vi "Client Init Test.vi"() -> (0 "no error":errorcluster, 1 "tags found":bool, 2 "expected execution settings":bool)   [LabVIEW 2013, in "OPC UA Server tests.lvlib"]
doc: "Tests Init override for server configuration"
uses:
  OPC UA Server tests.lvlib
  module/execution/OPC UA Server runtime.lvclass
  <vilib>/OPCUA/server/subVI/supported security policies.ctl
  module/configuration/OPC UA Server configuration.lvclass
  module/configuration/OPC UA Server configuration.lvclass/OPC UA Server configuration.ctl
  <vilib>/NI/Tag Bus/tag/tag descriptor.lvclass/tag descriptor.ctl
  <vilib>/NI/Tag Bus Module Framework/channel/TBM channel.lvclass/TBM channel.ctl
  <vilib>/NI/Tag Bus/tag/read tag name.vi
  <vilib>/NI/Tag Bus/tag/read data type.vi
  <vilib>/NI/Tag Bus Module Framework/channel/Read channel classification.vi
  module/configuration/Read Lines.vi
  <vilib>/NI/Tag Bus/dictionary/data dictionary.lvclass
  <vilib>/NI/Tag Bus Module Framework/channel/TBM channel.lvclass
  <vilib>/opcua/NI OPC UA Server.lvlib
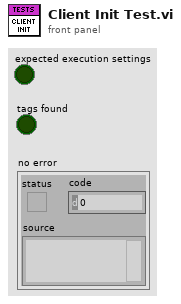
[diagram p1: front panel]
types:
  T1 = typedef "supported security policies.ctl" = cluster{"None":bool, "Sign with Basic128Rsa125":bool, "Sign and Encrypt with Basic128Rsa125":bool, "Sign with Basic256":bool, "Sign and Encrypt with Basic256":bool}
  T2 = cluster{"Client?":bool, "Server Certificates":cluster{"Relative Path?":bool, "Certificate Paths":path[], "Certificate Names":string[]}, "Client Certificates":cluster{"Relative Path?":bool, "Certificate Paths":path[], "Certificate Names":string[]}, "Client Configuration":cluster{"Server Endpoint URL":string, "Security Policy":cluster{"Message Mode":enum16{"None", "Sign", "Sign and Encrypt"}, "Security":enum16{"Basic256", "Basic128Rsa15"}}, "Username/Password":cluster{"Username":string, "Password":string}}, "Server Configuration":cluster{"Server Name":string, "TCP port (49580)":string, "Supported Security Policies":T1}}
  T3 = typedef "OPC UA configuration.lvclass/Line.ctl" = cluster{"channel":refnum<class "TBM channel.lvclass">, "Node Path":string, "OPC UA Data Type":T4}
  T4 = typedef "OPC UA configuration.lvclass/OPC UA Data Type.ctl" = u16
  T5 = typedef "TBM channel.lvclass/data tables.ctl" = cluster{"input data":T6, "processing parameter":T6, "processing result":T6, "output data":T6}
  T6 = typedef "tag bus.lvlib/dictionary table pair.ctl" = cluster{"data dictionary":refnum<class "data dictionary.lvclass">, "data table":T7}
  T7 = typedef "tag bus.lvlib/data table.lvlib/data table.ctl" = cluster{"Double":dbl[], "Single":sgl[], "I64":i64[], "I32":i32[], "I16":i16[], "I8":i8[], "U64":u64[], "U32":u32[], "U16":u16[], "U8":u8[], "Boolean":bool[], "String":string[], "Array of Double":cluster{"DBL Array":dbl[]}[], "Array of Single":cluster{"SGL Array":sgl[]}[], "Array of I64":cluster{"I64 Array":i64[]}[], "Array of I32":cluster{"I32 Array":i32[]}[], "Array of I16":cluster{"I16 Array":i16[]}[], "Array of I8":cluster{"I8 Array":i8[]}[], "Array of U64":cluster{"U64 Array":u64[]}[], "Array of U32":cluster{"U32 Array":u32[]}[], "Array of U16":cluster{"U16 Array":u16[]}[], "Array of U8":cluster{"U8 Array":u8[]}[], "Array of Boolean":cluster{"Boolean Array":bool[]}[], "Array of String":cluster{"String Array":string[]}[]}
  T8 = typedef "TBM module execution interface.lvclass/execution settings.ctl" = cluster{"reads inputs":bool, "processes data":bool, "writes outputs":bool}
  T9 = typedef "tag bus.lvlib/tag descriptor.lvclass/Data Type.ctl" = enum16{"Double", "Single", "I64", "I32", "I16", "I8", "U64", "U32", "U16", "U8", "Boolean", "String", "Array of Double", "Array of Single", "Array of I64", "Array of I32", "Array of I16", "Array of I8", "Array of U64", "Array of U32", "Array of U16", "Array of U8", "Array of Boolean", "Array of String"}
  T10 = typedef "TBM channel.lvclass/channel classification.ctl" = enum16{"input data", "output data", "processing parameter", "processing result"}
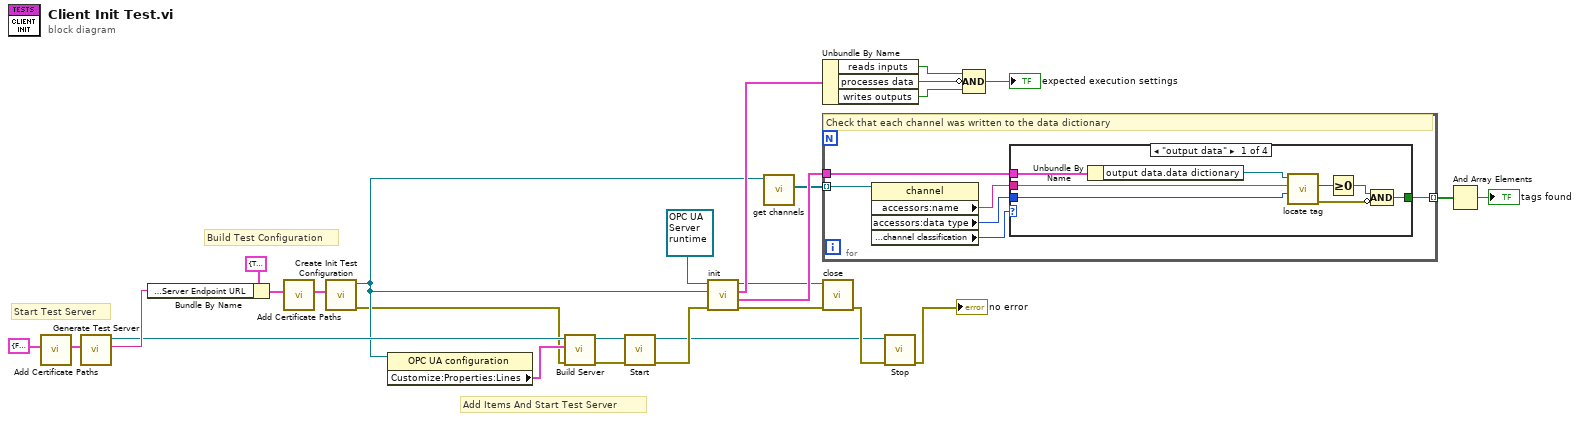
[diagram p0: block diagram]
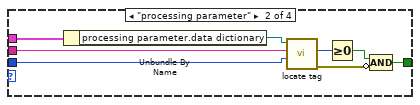
[diagram p2: hidden frame]
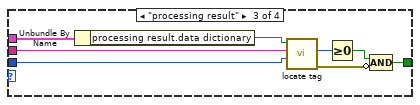
[diagram p3: hidden frame]
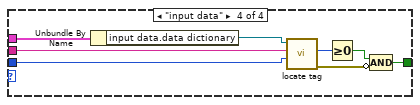
[diagram p4: hidden frame]
diagram:
  # "Add Items And Start Test Server"
  # "Start Test Server"
  # "Build Test Configuration"
  n1 = call "Add Certificate Paths.vi"("Connection Configuration in"=T2 {"Client?"=FALSE, "Server Certificates"={"Relative Path?"=FALSE, "Certificate Paths"=[path "C:/Users/Administrator/Desktop/OPC-UA-master/OPC-UA-master/Source/testing/Custom OPC UA Tests/Certificates/My Server.der"], "Certificate Names"=[]}, "Client Certificates"={"Relative Path?"=FALSE, "Certificate Paths"=[path "C:/Users/Administrator/Desktop/OPC-UA-master/OPC-UA-master/Source/testing/Custom OPC UA Tests/Certificates/DCAF Client Test Certificate.der"], "Certificate Names"=[]}, "Client Configuration"={"Server Endpoint URL"="", "Security Policy"={"Message Mode"=enum."None", "Security"=enum."Basic256"}, "Username/Password"={"Username"="", "Password"=""}}, "Server Configuration"={"Server Name"="Test", "TCP port (49580)"="49580", "Supported Security Policies"={"None"=TRUE, "Sign with Basic128Rsa125"=FALSE, "Sign and Encrypt with Basic128Rsa125"=FALSE, "Sign with Basic256"=FALSE, "Sign and Encrypt with Basic256"=FALSE}}} ("Connection Configuration")) -> ("Connection Configuration out"=w12:T2)  [unwired: 10 in]
  n2 = call "Generate Test Server.vi"("Connection Configuration"=w12) -> ("OPC UA server refnum out"=w10:refnum<k21>, "server endpoint URL"=w11:string)  [unwired: 7 in, 1 out]
  n3 = Bundle By Name(cluster=T2 {"Client?"=TRUE, "Server Certificates"={"Relative Path?"=FALSE, "Certificate Paths"=[path "C:/Users/Administrator/Desktop/OPC-UA-master/OPC-UA-master/Source/testing/Custom OPC UA Tests/Certificates/My Server.der"], "Certificate Names"=[]}, "Client Certificates"={"Relative Path?"=FALSE, "Certificate Paths"=[path "C:/Users/Administrator/Desktop/OPC-UA-master/OPC-UA-master/Source/testing/Custom OPC UA Tests/Certificates/DCAF Client Test Certificate.der"], "Certificate Names"=[]}, "Client Configuration"={"Server Endpoint URL"="", "Security Policy"={"Message Mode"=enum."None", "Security"=enum."Basic256"}, "Username/Password"={"Username"="", "Password"=""}}, "Server Configuration"={"Server Name"="Test", "TCP port (49580)"="49580", "Supported Security Policies"={"None"=TRUE, "Sign with Basic128Rsa125"=FALSE, "Sign and Encrypt with Basic128Rsa125"=FALSE, "Sign with Basic256"=FALSE, "Sign and Encrypt with Basic256"=FALSE}}} ("Connection Configuration"), "Client Configuration.Server Endpoint URL"=w11) -> (w15:T2)
  n4 = call "Add Certificate Paths.vi"("Connection Configuration in"=w15) -> ("Connection Configuration out"=w17:T2)  [unwired: 10 in]
  n5 = call "Create Init Test Configuration.vi"("Connection Configuration"=w17) -> ("error out"=w7:errorcluster, "module"=w9:refnum<class "OPC UA Server configuration.lvclass">)  [unwired: 9 in]
  n6 = property class="OPC UA configuration"(reference=w9) -> ("Customize:Properties:Lines"=w8:T3[])  [unwired: 1 in, 2 out]
  n7 = call "Build Server.vi"("Error In"=w7, "Lines"=w8, "OPC UA server refnum in"=w10) -> ("Error Out"=w6:errorcluster, "OPC UA server refnum out"=w2:refnum<k21>)  [unwired: 7 in]
  n8 = call <vilib>:"Start.vi"("error in (no error)"=w6, "OPC UA server refnum in"=w2) -> ("error out"=w3:errorcluster, "OPC UA server refnum out"=w1:refnum<k21>)  [unwired: 8 in]
  n9 = call-dynamic "init.vi"("error in"=w3, "TBM module configuration in"=w9, "OPC UA runtime in"=refnum<class "OPC UA Server runtime.lvclass"> refnum ("tag bus configurable plugin module")) -> ("error out"=w20:errorcluster, "data allocations"=w28:T5, "execution settings"=w27:T8, "OPC UA runtime out"=w14:refnum<class "OPC UA Server runtime.lvclass">)  [unwired: 5 in]
  n10 = call-dynamic "get channels.vi"("OPC UA configuration in"=w9) -> ("channels"=w18:refnum<class "TBM channel.lvclass">[])  [unwired: 9 in, 1 out]
  n11 = Unbundle By Name(w27) -> ("reads inputs"=w26:bool, "processes data"=w24:bool, "writes outputs"=w25:bool)
  n12 = for {
    tunnel: w28 -> [w34]
    tunnel: w18 -> [w33] mode=indexing
    tunnel: [w32] -> w22 mode=indexing
    # "Check that each channel was written to the data dictionary"
    n13 = property class="channel"(reference=w33) -> ("accessors:name"=w29:string, "accessors:data type"=w30:T9, "data access:channel classification"=w31:T10)  [unwired: 1 in, 2 out]
    n14 = case shown="\"output data\"" w31 {
      tunnel: w34 -> [w42 w50 w58 w66]
      tunnel: w30 -> [w40 w48 w56 w64]
      tunnel: w29 -> [w39 w47 w55 w63]
      tunnel: [w35 w43 w51 w59] -> w32
      frame "output data" {
        n15 = Unbundle By Name(w42) -> ("output data.data dictionary"=w41:refnum<class "data dictionary.lvclass">)
        n16 = call <vilib>:"locate tag.vi"("data type"=w40, "name"=w39, "data dictionary in"=w41) -> ("error out"=w36:errorcluster, "index"=w38:i32)  [unwired: 6 in, 1 out]
        n17 = Greater Or Equal To 0?(x=w38) -> (x >= 0?=w37:bool)
        n18 = Compound Arithmetic op=AND(w37, invert w36) -> (w35:bool)
      }
      frame "processing parameter" {
        n19 = Unbundle By Name(w50) -> ("processing parameter.data dictionary"=w49:refnum<class "data dictionary.lvclass">)
        n20 = call <vilib>:"locate tag.vi"("data type"=w48, "name"=w47, "data dictionary in"=w49) -> ("error out"=w44:errorcluster, "index"=w46:i32)  [unwired: 6 in, 1 out]
        n21 = Greater Or Equal To 0?(x=w46) -> (x >= 0?=w45:bool)
        n22 = Compound Arithmetic op=AND(w45, invert w44) -> (w43:bool)
      }
      frame "processing result" {
        n23 = Unbundle By Name(w58) -> ("processing result.data dictionary"=w57:refnum<class "data dictionary.lvclass">)
        n24 = call <vilib>:"locate tag.vi"("data type"=w56, "name"=w55, "data dictionary in"=w57) -> ("error out"=w52:errorcluster, "index"=w54:i32)  [unwired: 6 in, 1 out]
        n25 = Greater Or Equal To 0?(x=w54) -> (x >= 0?=w53:bool)
        n26 = Compound Arithmetic op=AND(w53, invert w52) -> (w51:bool)
      }
      frame "input data" {
        n27 = Unbundle By Name(w66) -> ("input data.data dictionary"=w65:refnum<class "data dictionary.lvclass">)
        n28 = call <vilib>:"locate tag.vi"("data type"=w64, "name"=w63, "data dictionary in"=w65) -> ("error out"=w60:errorcluster, "index"=w62:i32)  [unwired: 6 in, 1 out]
        n29 = Greater Or Equal To 0?(x=w62) -> (x >= 0?=w61:bool)
        n30 = Compound Arithmetic op=AND(w61, invert w60) -> (w59:bool)
      }
    }
  }
  n31 = call-dynamic "close.vi"("error in"=w20, "OPC UA runtime in"=w14) -> ("error out"=w5:errorcluster)  [unwired: 9 in]
  n32 = call <vilib>:"Stop.vi"("error in (no error)"=w5, "OPC UA server refnum in"=w1) -> ("error out"=→"no error":errorcluster)  [unwired: 8 in, 1 out]
  n33 = Compound Arithmetic op=AND(w26, invert w24, w25) -> (→"expected execution settings":bool)
  n34 = And Array Elements(Boolean array=w22) -> (logical AND=→"tags found":bool)
